vi "test double slider window control.vi"() -> ()   [LabVIEW 2025]
uses:
  <vilib>/numeric/Random Number (Range) U64.vi
  <vilib>/numeric/sub_Random U32.vi
panel:
  out "slider 0":u32
  out "slider 1":u32
  in  "stop":bool
  in  "Slide":cluster{u32, u32}(slide)={0, 10} scale=0.0..1063.0
  out "Image":T1(plugin-control)
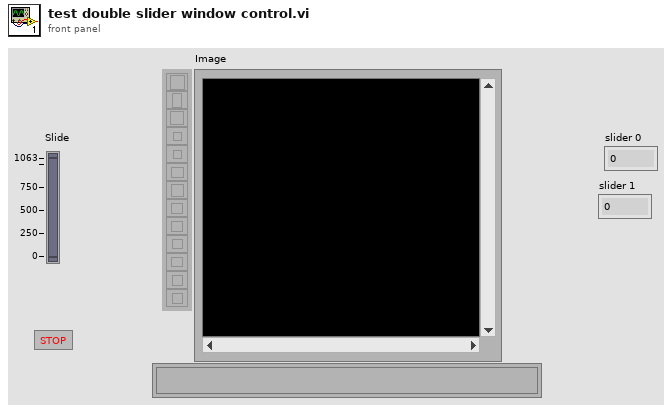
[diagram p1: front panel]
types:
  T1 = typedef "IMAQ Image.ctl" = refnum<image>
  T2 = typedef "Image Type" = u32
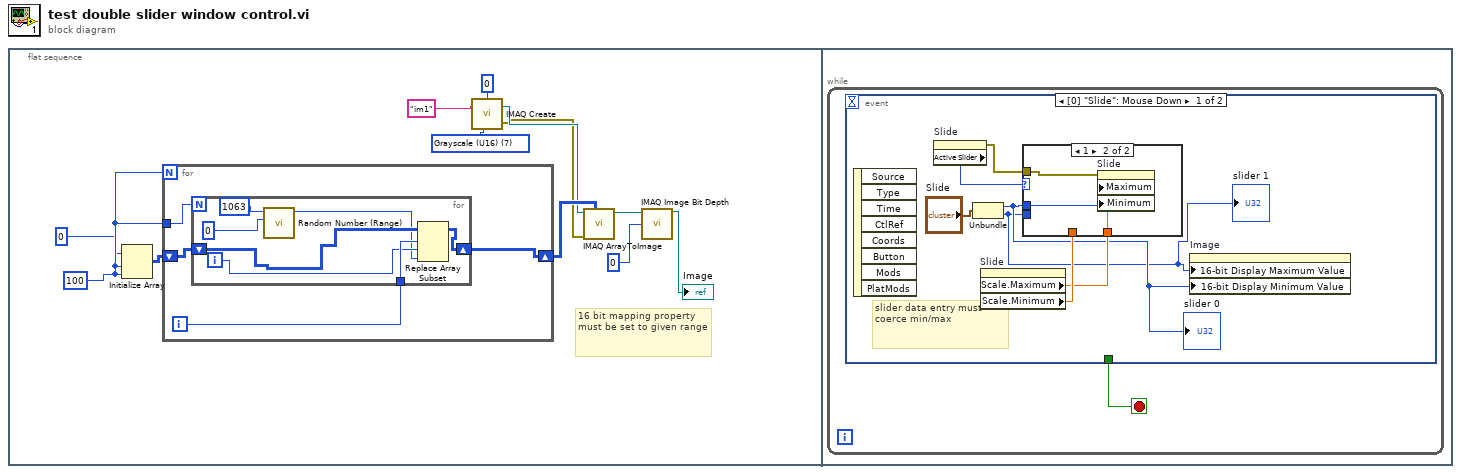
[diagram p0: block diagram]
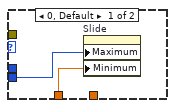
[diagram p2: hidden frame]
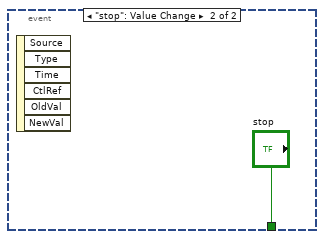
[diagram p3: hidden frame]
diagram:
  n1 = flat-sequence {
    frame #0 {
      w6 = T2 7 items=["Grayscale (U8)", "Grayscale (I16)", "Grayscale (SGL)", "Complex (CSG)", "RGB (U32)", "HSL (U32)", "RGB (U64)", "Grayscale (U16)"] ("Image Type")
      w12 = 100 ("dimension size")
      # "16 bit mapping property must be set to given range"
      n2 = Initialize Array(u64 0 ("element"), w12, w12) -> (w11:u64[][])
      n3 = for {
        N: w12 -> [_]
        tunnel: w12 -> [w16]
        shift-right: [w14] -> w9
        shift-left: w11 -> [w15]
        i -> [w13]
        n4 = for {
          N: w16 -> [_]
          shift-right: [w17] -> w14
          shift-left: w15 -> [w21]
          tunnel: w13 -> [w20]
          i -> [w19]
          n5 = call-poly <vilib>:"Random Number (Range).vi"("lower bound (0)"=u64 0, "upper bound (100)"=u64 1063) -> ("number"=w18:u64)  [unwired: 9 in]
          n6 = Replace Array Subset(array=w21, new element=w18, index (row)=w20, index (col)=w19) -> (w17:u64[][])
        }
      }
      n7 = call "IMAQ Create"("Border Size"=0, "Image Name"="im1", "Image Type"=w6) -> ("New Image"=w8:T1, "error out"=w7:errorcluster)  [unwired: 2 in]
      n8 = call "IMAQ ArrayToImage"("Image Pixels (U16)"=w9, "error in (no error)"=w7, "Image"=w8) -> ("Image Out"=w2:T1)  [unwired: 7 in, 1 out]
      n9 = call "IMAQ Image Bit Depth"("Image"=w2, "Bit Depth (0)"=u32 0) -> ("Image Out"=→"Image":T1)  [unwired: 11 in, 2 out]
    }
    frame #1 {
      n10 = while {
        stop <- w24 stop-if-true
        n11 = event shown="[0] \"Slide\": Mouse Down" {
          selector: _ -> [_ _]
          dyn-events: _ -> [_ _]
          timeout: _ -> [_ _]
          tunnel: [_ "stop"] -> w24
          event "Slide": Mouse Down {
            # "slider data entry must coerce min/max"
            n12 = event-data() -> ()  [unwired: 1 in, 8 out]
            n13 = property on="Slide" class="Slide (strict)"() -> (error out=w30:errorcluster, "Active Slider"=w29:i32)  [unwired: 2 in, 1 out]
            n14 = Unbundle("Slide") -> (w26:u32, w25:u32)
            "slider 1" <- w25
            "slider 0" <- w26
            n15 = property on="Slide" class="Slide (strict)"() -> ("Scale.Maximum"=w27:dbl, "Scale.Minimum"=w28:dbl)  [unwired: 2 in, 2 out]
            n16 = case shown="1" w29 {
              tunnel: w30 -> [_ w36]
              tunnel: w28 -> [w33 _]
              tunnel: w25 -> [w32 _]
              tunnel: w27 -> [_ w35]
              tunnel: w26 -> [_ w34]
              frame 0, Default {
                n17 = property on="Slide" class="Slide (strict)"("Maximum"=w32, "Minimum"=w33) -> ()  [unwired: 2 in, 2 out]
              }
              frame 1 {
                n18 = property on="Slide" class="Slide (strict)"(error in=w36, "Maximum"=w35, "Minimum"=w34) -> ()  [unwired: 1 in, 2 out]
              }
            }
            n19 = property on="Image" class="ImageControl"("16-bit Display Maximum Value"=w25, "16-bit Display Minimum Value"=w26) -> ()  [unwired: 2 in, 2 out]
          }
          event "stop": Value Change {
            n20 = event-data() -> ()  [unwired: 1 in, 6 out]
          }
        }
      }
    }
  }
